vi "GetADSPathsForTwinCAT.vi"() -> ()   [LabVIEW 2022 SP3]
uses:
  <userlib>/Beckhoff-LabVIEW-Interface/_DependsOn/TypeDefs/Low-Levels/Symbol Interface Mode.ctl
  <userlib>/Beckhoff-LabVIEW-Interface/_DependsOn/TypeDefs/Utilities/License State.ctl
panel:
  out "LicenseState":T1[](array[typedef])
  out "WriteGrpSymbols":string[](array[string])
  out "ReadGrpSymbols":string[](array[string])
  out "List of Registered Targets":string[](array[string])
  out "PortInfo":string
  in  "Symbol Interface Mode":T2=enum."Read & Write"
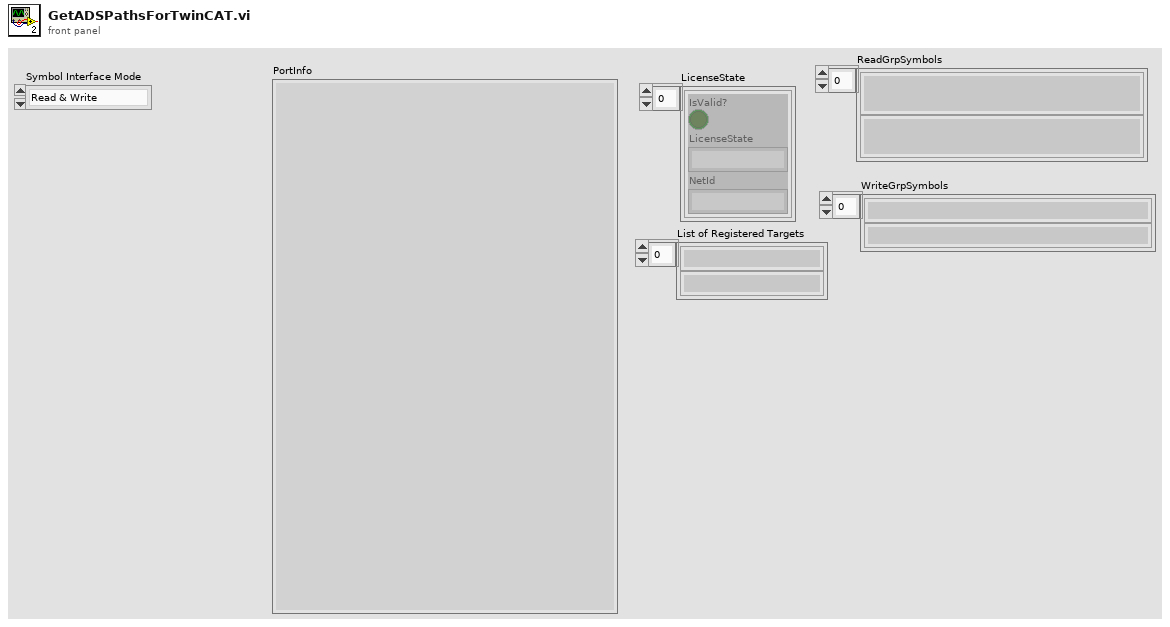
[diagram p1: front panel]
types:
  T1 = typedef "License State.ctl" = cluster{"IsValid?":bool, "LicenseState":string, "NetId":string}
  T2 = typedef "Symbol Interface Mode.ctl" = enum16{"Read Only", "Write Only", "Read & Write"}
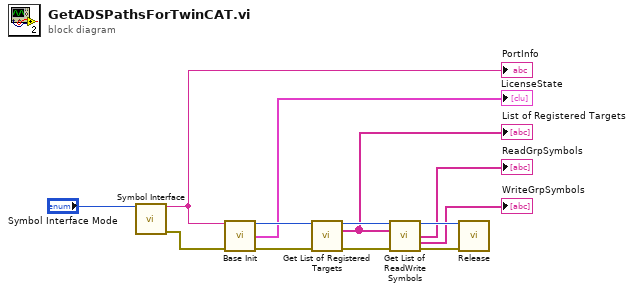
[diagram p0: block diagram]
diagram:
  n1 = call <userlib>:"Symbol Interface.vi"("Symbol Interface Mode"="Symbol Interface Mode") -> ("PortInfo"=w3:string, "error out"=w2:errorcluster)  [unwired: 13 in]
  "PortInfo" <- w3
  n2 = call <userlib>:"Base Init .vi"("XMLDescription"=w3, "error in (no error)"=w2) -> ("Handle"=w7:u32, "LicenseState"=→"LicenseState":T1[], "error out"=w6:errorcluster)  [unwired: 11 in]
  n3 = call <userlib>:"Get List of Registered Targets.vi"("Handle"=w7, "error in (no error)"=w6) -> ("Handle"=w12:u32, "List of Registered Targets"=w11:string[], "error out"=w9:errorcluster)  [unwired: 11 in]
  "List of Registered Targets" <- w11
  n4 = call <userlib>:"Get List of ReadWrite Symbols.vi"("Handle"=w12, "List of Registered Targets"=w11, "error in (no error)"=w9) -> ("Handle"=w10:u32, "ReadGrpSymbols"=→"ReadGrpSymbols":string[], "WriteGrpSymbols"=→"WriteGrpSymbols":string[], "error out"=w8:errorcluster)  [unwired: 9 in]
  n5 = call <userlib>:"Release.vi"("Handle"=w10, "error in (no error)"=w8) -> ()  [unwired: 13 in, 1 out]
